vi "MTMount_putSample_ElevationDrives.vi"(8 "error in (no error)":errorcluster, 11 "Elevation_Drives_Ctl":T1) -> (0 "error out":errorcluster, 2 "function return":i32, 3 "Elevation_Drives_Ctl out":T1)   [LabVIEW 2018, in "SALLV_MTMount.lvlib"]
doc: "int MTMount_shm_putSample_Elevation_DrivesLV(MTMount_Elevation_DrivesLV *Elevation_Drives_Ctl );"
uses:
  SALLV_MTMount.lvlib
  DataTypes/Elevation_Drives.ctl
  SALLV_MTMount.so
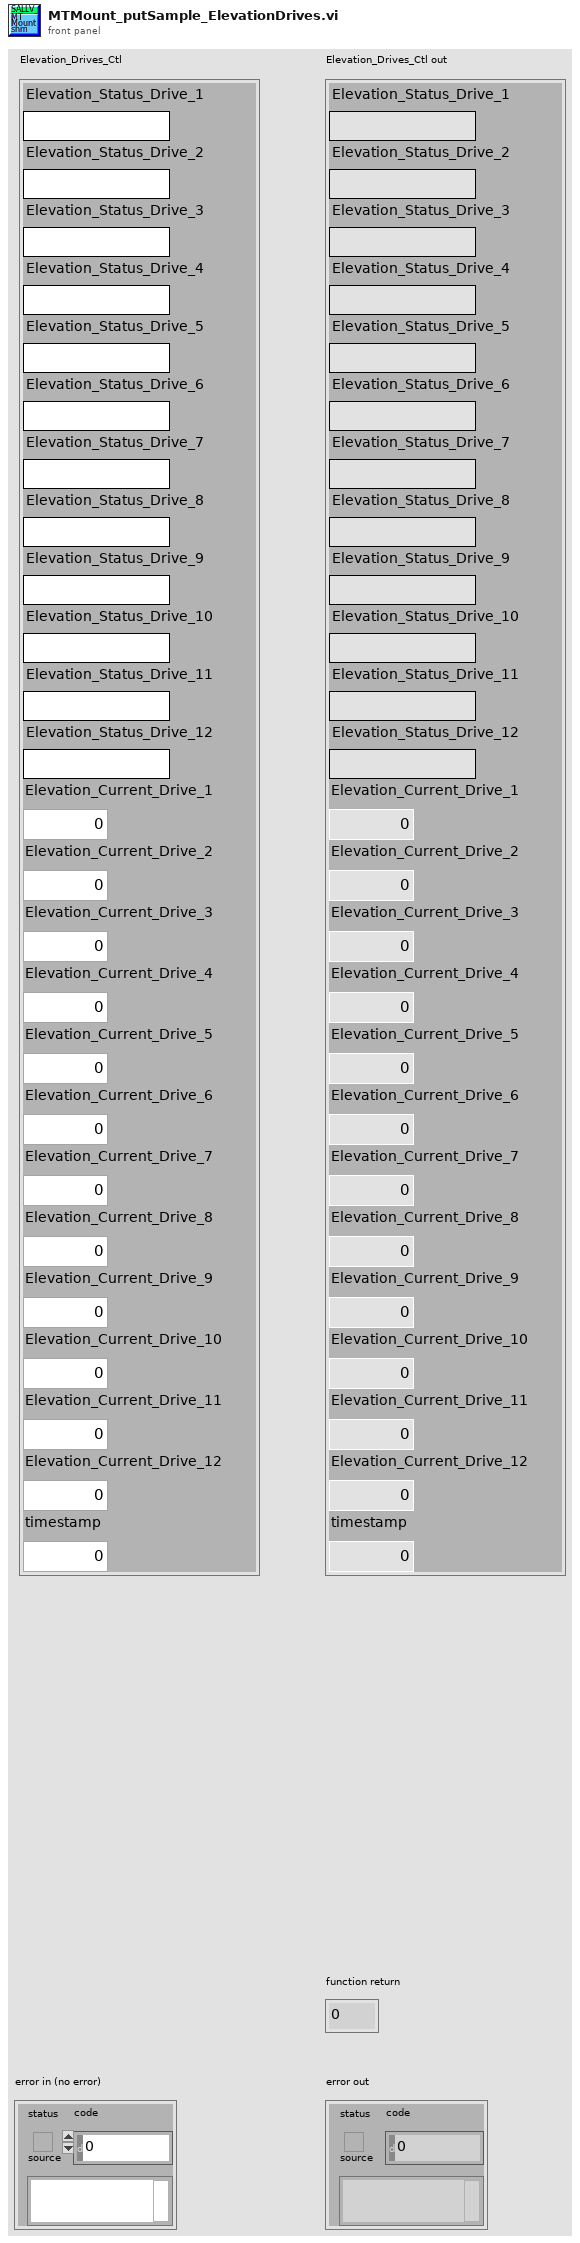
[diagram p1: front panel]
types:
  T1 = typedef "SALLV_MTMount.lvlib/Elevation_Drives.ctl" = cluster{"Elevation_Status_Drive_1":string, "Elevation_Status_Drive_2":string, "Elevation_Status_Drive_3":string, "Elevation_Status_Drive_4":string, "Elevation_Status_Drive_5":string, "Elevation_Status_Drive_6":string, "Elevation_Status_Drive_7":string, "Elevation_Status_Drive_8":string, "Elevation_Status_Drive_9":string, "Elevation_Status_Drive_10":string, "Elevation_Status_Drive_11":string, "Elevation_Status_Drive_12":string, "Elevation_Current_Drive_1":dbl, "Elevation_Current_Drive_2":dbl, "Elevation_Current_Drive_3":dbl, "Elevation_Current_Drive_4":dbl, "Elevation_Current_Drive_5":dbl, "Elevation_Current_Drive_6":dbl, "Elevation_Current_Drive_7":dbl, "Elevation_Current_Drive_8":dbl, "Elevation_Current_Drive_9":dbl, "Elevation_Current_Drive_10":dbl, "Elevation_Current_Drive_11":dbl, "Elevation_Current_Drive_12":dbl, "timestamp":dbl}
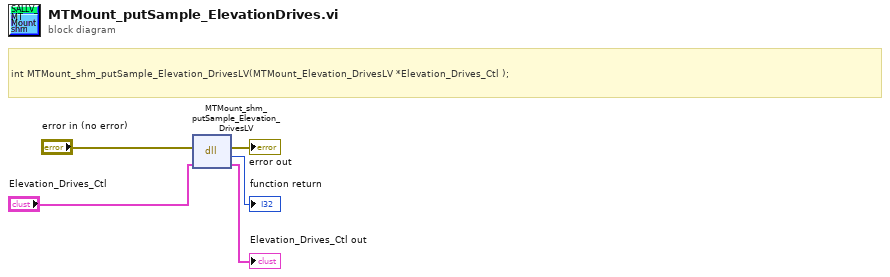
[diagram p0: block diagram]
diagram:
  # "int MTMount_shm_putSample_Elevation_DrivesLV(MTMount_Elevation_DrivesLV *Elevation_Drives_Ctl );"
  n1 = dll-call lib="home/ttsai/Document/salApiMTMount/SALLV_MTMount/SALLV_MTMount.*" fn="MTMount_shm_putSample_Elevation_DrivesLV"(error in="error in (no error)", "Elevation_Drives_Ctl"="Elevation_Drives_Ctl") -> (error out=→"error out":errorcluster, →"function return":i32, "Elevation_Drives_Ctl"=→"Elevation_Drives_Ctl out":T1)  [unwired: 2 in, 1 out]
